vi "ep_Y to D convert (Vector).vi"(8 "error in (no error)":errorcluster, 11 "one-cycle fundamental phase voltage vectors":T2(array[cluster])) -> (0 "error out":errorcluster, 3 "one-cycle fundamental line voltage vectors":T2(array[cluster]))   [LabVIEW 2014, in "NI_EP_Power Quality.lvlib"]
uses:
  <vilib>/addons/Electrical Power/PQ/NI_EP_Power Quality.lvlib
  <vilib>/addons/Electrical Power/PQ/Common/Controls/ep_AI Data Channel.ctl
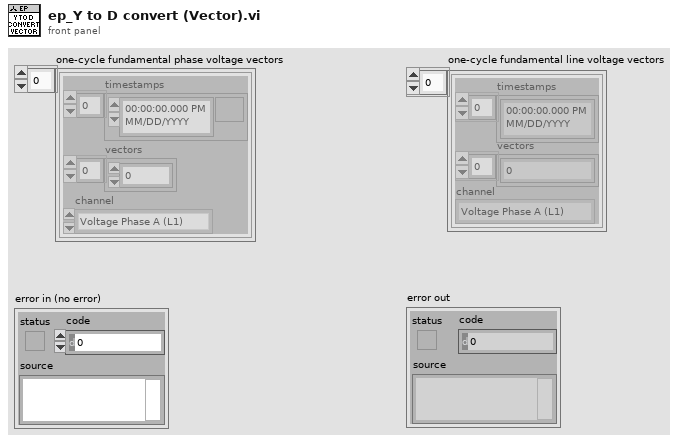
[diagram p1: front panel]
types:
  T1 = typedef "NI_EP_Power Quality.lvlib/ep_AI Data Channel.ctl" = enum16{"Voltage Phase A (L1)", "Voltage Phase B (L2)", "Voltage Phase C (L3)", "Voltage Phase N (Neutral)", "Current Phase A (L1)", "Current Phase B (L2)", "Current Phase C (L3)", "Current Phase N (Neutral)"}
  T2 = cluster{"timestamps":timestamp[], "vectors":cdb[], "channel":T1}[]
  T3 = cluster{"timestamps":timestamp[], "vectors":cdb[], "channel":T1}
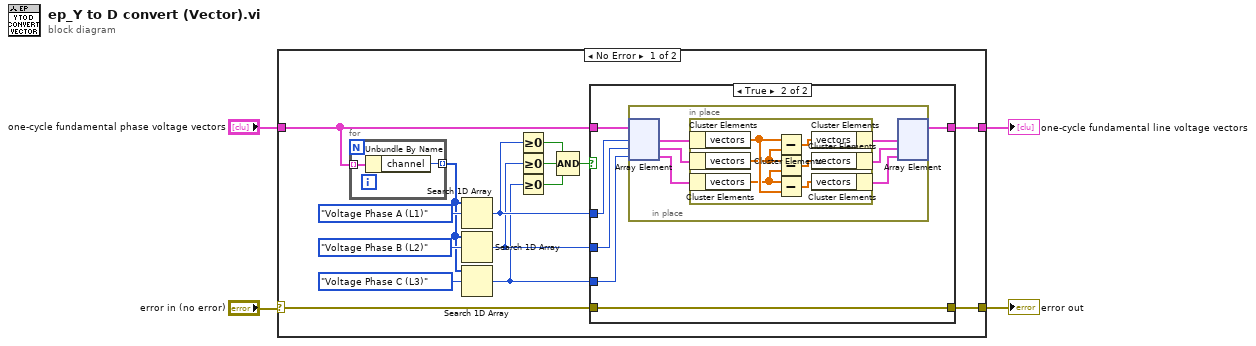
[diagram p0: block diagram]
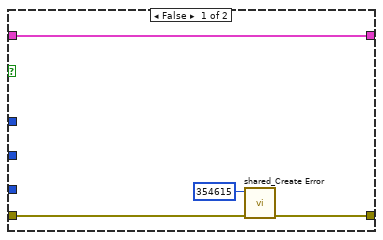
[diagram p2: hidden frame]
diagram:
  n1 = case shown="No Error" "error in (no error)" {
    selector: "error in (no error)" -> [w6 w44]
    tunnel: [w19 _] -> w4
    tunnel: "one-cycle fundamental phase voltage vectors" -> [w18 _]
    tunnel: [w5 w44] -> w1
    frame No Error {
      n2 = for {
        tunnel: w18 -> [w43] mode=indexing
        tunnel: [w42] -> w13 mode=indexing
        n3 = Unbundle By Name(w43) -> ("channel"=w42:T1)
      }
      n4 = Search 1D Array(1D array=w13, element=ep_AI_Data_Channel."Voltage Phase A (L1)" ("AI data channel")) -> (index of element=w9:i32)  [unwired: 1 in]
      n5 = Search 1D Array(1D array=w13, element=ep_AI_Data_Channel."Voltage Phase B (L2)" ("AI data channel")) -> (index of element=w8:i32)  [unwired: 1 in]
      n6 = Search 1D Array(1D array=w13, element=ep_AI_Data_Channel."Voltage Phase C (L3)" ("AI data channel")) -> (index of element=w7:i32)  [unwired: 1 in]
      n7 = Greater Or Equal To 0?(x=w9) -> (x >= 0?=w17:bool)
      n8 = Greater Or Equal To 0?(x=w8) -> (x >= 0?=w12:bool)
      n9 = Greater Or Equal To 0?(x=w7) -> (x >= 0?=w11:bool)
      n10 = Compound Arithmetic op=AND(w17, w12, w11) -> (w10:bool)
      n11 = case shown="True" w10 {
        tunnel: [w23 w25] -> w19
        tunnel: w18 -> [w23 w29]
        tunnel: w9 -> [_ w28]
        tunnel: w8 -> [_ w27]
        tunnel: w7 -> [_ w26]
        tunnel: w6 -> [w21 w24]
        tunnel: [w20 w24] -> w5
        frame False {
          n12 = call <vilib>:"shared_Create Error.vi"("error in (no error)"=w21, "error code (0)"=354615) -> ("error out"=w20:errorcluster)  [unwired: 9 in]
        }
        frame True {
          n13 = in-place {
            n14 = in-place-array #1(w29, w28, w27, w26) -> (w35:T3, w34:T3, w33:T3)
            n15 = in-place {
              n16 = in-place-cluster #2(w35) -> ("vectors"=w41:cdb[])
              n17 = in-place-cluster #3(w34) -> ("vectors"=w40:cdb[])
              n18 = in-place-cluster #4(w33) -> ("vectors"=w39:cdb[])
              n19 = Subtract(x=w41, y=w40) -> (x-y=w36:cdb[])
              n20 = Subtract(x=w40, y=w39) -> (x-y=w37:cdb[])
              n21 = Subtract(x=w39, y=w41) -> (x-y=w38:cdb[])
              n22 = in-place-cluster #2("vectors"=w36) -> (w32:T3)
              n23 = in-place-cluster #3("vectors"=w37) -> (w31:T3)
              n24 = in-place-cluster #4("vectors"=w38) -> (w30:T3)
            }
            n25 = in-place-array #1(w32, w31, w30) -> (w25:T2)  [unwired: 3 out]
          }
        }
      }
    }
    frame Error {
    }
  }
  "one-cycle fundamental line voltage vectors" <- w4
  "error out" <- w1
